vi "Init.vi"(8 "error in (no error)":errorcluster, 10 "Default Index File (index.html)":string="index.html", 11 "Public Root":path) -> (0 "error out":errorcluster, 3 "StandardFileServe out":refnum<class "StandardFileServe.lvclass">)   [LabVIEW 2020, in "HTTP Server.lvlib" / "StandardFileServe.lvclass"]
doc: "Initializes the capability of serving files directly from disk within a root folder. Allows specifying a default filename to provide when the requested path is a folder. (For instance, when requesting the root path /, the index.html would be served from the Public Root folder without needing to specify /index.html explicitly in the URL.\n\nThis controller will serve any file requested within the Public Root folder and all subfolders and there is no custom file filtering so ensure no private files exist under the Public Root folder. If access is required to portions of protected files, for instance, a custom controller can be implemented that can access specific files anywhere on the system. \n\nThe content-type header for known file extensions will be set automatically. The content-type mime table exists in the HTTP Utils package."
uses:
  StandardFileServe.lvclass
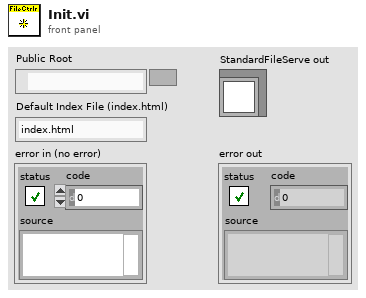
[diagram p1: front panel]
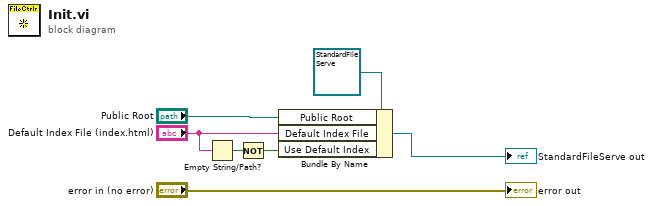
[diagram p0: block diagram]
diagram:
  n1 = Empty String/Path?(string/path="Default Index File (index.html)") -> (empty?=w2:bool)
  n2 = Not(x=w2) -> (.not. x?=w1:bool)
  n3 = Bundle By Name(cluster=refnum<class "StandardFileServe.lvclass"> refnum ("StandardFileServe out"), "Public Root"="Public Root", "Default Index File"="Default Index File (index.html)", "Use Default Index"=w1) -> (→"StandardFileServe out":refnum<class "StandardFileServe.lvclass">)
  "error out" <- "error in (no error)"
